vi "SCT Localization Strings.vi"() -> ()   [LabVIEW 2016]
panel:
  in  "Invalid Custom Data Type Error Message":string="数据类型无效。编辑自定义控件文件可解决问题。数据类型将还原至以前的设置。" caption="无效自定义数据类型错误信息"
  in  "Revert":string="还原" caption="还原"
  in  "Apply":string="应用" caption="应用"
  in  "Spreadsheet Click Apply/Revert":string="当前所选共享变量已被修改，但未应用这些改动。是否应用改动？" caption="电子表格单击应用/还原"
  in  "Library open in project":string="在项目中已打开该库。编辑器将配置内存中的库实例。" caption="项目中打开的库"
  in  "Failed to get path for feature pack":string="无法获取%s的路径。\n\n%s" caption="无法获取功能包的路径"
  in  "Failed to start feature pack":string="无法开始%s。\n\n%s" caption="无法启动功能包"
  in  "VarMan::Network Variable Bind to Source Message":string="该变量的源绑定已更改为网络URL，而不是项目项。" caption="VarMan::网络变量数据源绑定的信息"
  in  "Incompatible Custom Data Type Error Message":string="该数据类型对已有变量配置无效。数据类型将还原至以前的设置。" caption="不兼容自定义数据类型错误信息"
  in  "Corrupt Message":string="部分变量配置已损坏并被设置为默认值。" caption="损坏信息"
  in  "Cancel":string="取消" caption="取消"
  in  "Continue":string="继续" caption="继续"
  in  "Uninstalled Feature Packs Message":string="该项目的部分已启用选项不适用于本计算机。如未安装所需模块，通常将导致选项不可用。如继续编辑共享变量的属性，共享变量属性对话框中以下页面的选项将被禁用:\n\n%s\n\n是否继续？" caption="未安装功能包信息"
  in  "Format string":string="启用%s" caption="格式字符串"
  in  "Init Category Val":string="变量" caption="初始类别值"
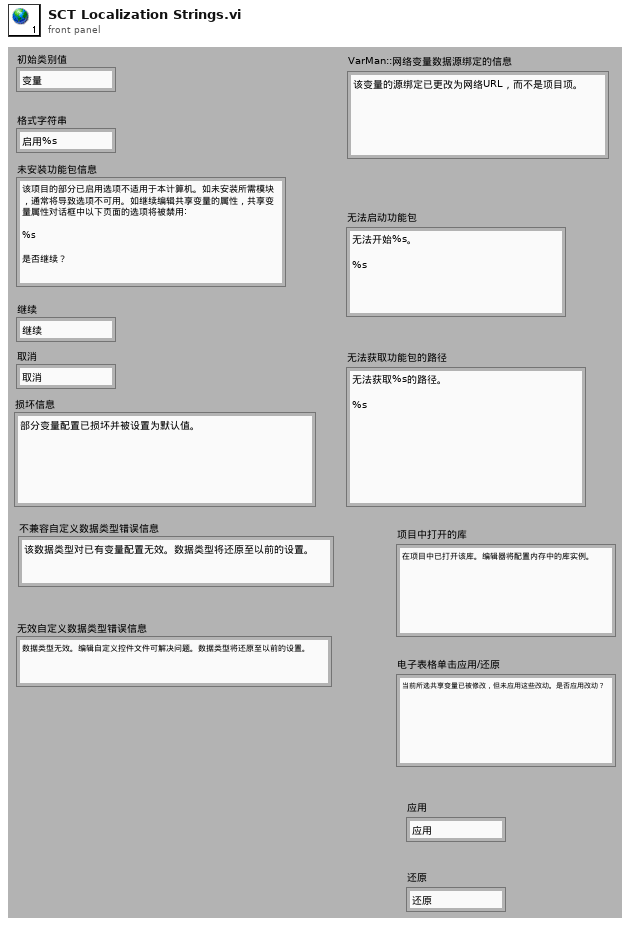
[diagram p1: front panel]
diagram:
